vi "Test Communication between PXG5 and DAQ Device.vi"() -> ()   [LabVIEW 2021]
panel:
  out "Analog In (ai0) [0-100%]":dbl format="%.2g"
  in  "Stop Button":bool
  out "Analog In (ai0) [0-5V]":dbl format="%.2g"
  in  "Analog Out (ao0) [1-5V]":dbl=1.0 min=1.0 max=5.0 step=0.1 format="%.2g"
  # "Process Variable (PV) in Voltage [1-5V]. Depending on the settings on the PXG5, you will se Voltage or in Engineering Unit [°C], either 20-50°C or 0-50°C depending on your settings"
  # "PV"
  # "Manipulated Value (MV) in Voltage [0-5V]. \nOn the PXG5, you will set MV between 0-100%"
  # "MV"
  # "MV"
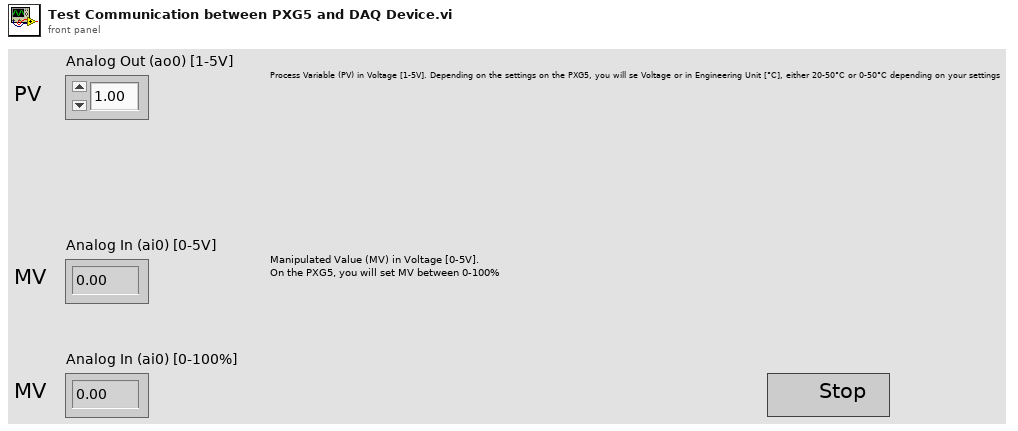
[diagram p1: front panel]
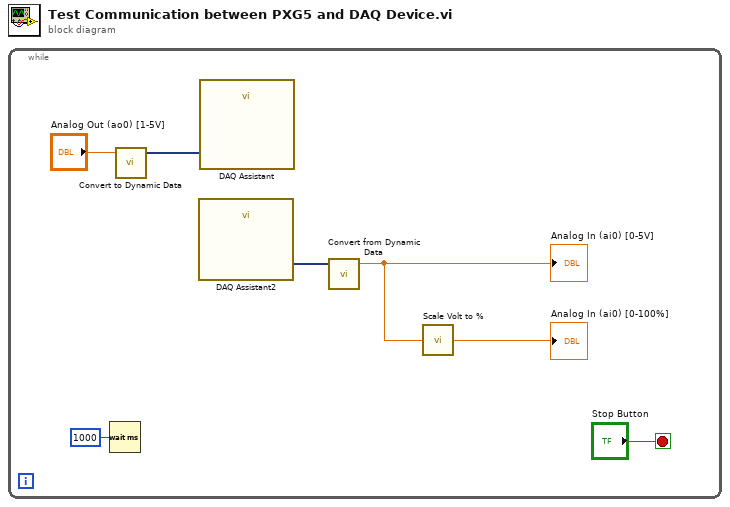
[diagram p0: block diagram]
diagram:
  n1 = while {
    stop <- "Stop Button" stop-if-true
    n2 = Wait (ms)(milliseconds to wait=u32 1000) -> ()  [unwired: 1 out]
    n3 = call "Convert to Dynamic Data"("Double"="Analog Out (ao0) [1-5V]") -> ("Dynamic Data Type"=w3:dynamicdata)  [unwired: 3 in]
    n4 = call "DAQ Assistant2"() -> ("data"=w5:dynamicdata)  [unwired: 17 in, 2 out]
    n5 = call "DAQ Assistant"("data"=w3) -> ()  [unwired: 17 in, 2 out]
    n6 = call "Convert from Dynamic Data"("Dynamic Data Type"=w5) -> ("Scalar"=w2:dbl)  [unwired: 3 in]
    "Analog In (ai0) [0-5V]" <- w2
    n7 = call "Scale Volt to %.vi"("Input Value [0-5V]"=w2) -> ("Output Value [0-100%]"=→"Analog In (ai0) [0-100%]":dbl)
  }
